vi "Prax12.3.4.vi"() -> ()   [LabVIEW 2020]
uses:
  Prax12.3.1.vi
panel:
  out "Array":dbl[](array[numeric])=[3.0, 2.0, 5.0, 8.0, 1.0]
  out "transposed array":dbl[][](array[numeric])
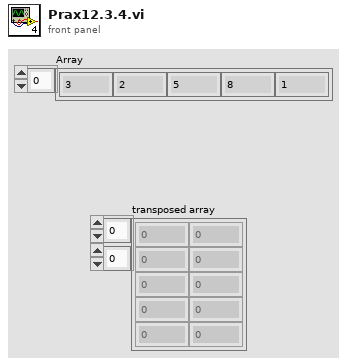
[diagram p1: front panel]
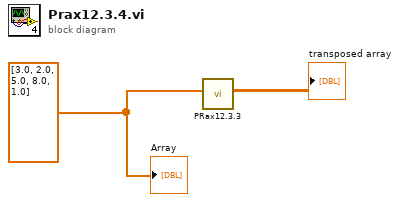
[diagram p0: block diagram]
diagram:
  w1 = dbl[] [3.0, 2.0, 5.0, 8.0, 1.0]
  n1 = call-poly "PRax12.3.3.vi"("Array"=w1) -> ("transposed array"=→"transposed array":dbl[][])  [unwired: 10 in]
  "Array" <- w1
